vi "Begin.vi"() -> (0 "error out":errorcluster)   [LabVIEW 2013]
doc: "Called before other user functions, this VI is expected to open initial I/O refnums, load in file data, and do all program initialization. Notice that the <B>error out</B> terminal is simply used for data flow. Wiring it to other structures or subVIs ensures that this VI runs first."
uses:
  <vilib>/Rock Robotics/WPI/DriverStation/WPI_DriverStationRobotMode2.ctl
  <vilib>/Rock Robotics/WPI/Joystick/WPI_JoystickDeviceEnum.ctl
  <vilib>/Rock Robotics/WPI/SafetyOutput/WPI_SafetyOutputConfigMenu.ctl
  <vilib>/Rock Robotics/SystemInterfaces/DIO/FPGA_DIOPWMChannel.ctl
  Robot Global Data.vi
  <vilib>/Utility/config.llb/Read Key (Double).vi
  <vilib>/Utility/config.llb/Read Key (String).vi
  <vilib>/Rock Robotics/WPI/RobotDrive/WPI_RobotDriveOpen2MotorWithJaguar.vi
  <vilib>/Rock Robotics/WPI/MotorControl/WPI_MotorControlOpen Jaguar.vi
  <vilib>/Rock Robotics/SystemInterfaces/Typedef/FPGA_TypedefDigitalModule.ctl
  <vilib>/Rock Robotics/WPI/CAN/Jaguar/SubVIs/WPI_CANJaguar_ControlMode.ctl
  <vilib>/Rock Robotics/WPI/MotorControl/WPI_MotorControlOpenCANJaguar.vi
  <vilib>/Utility/config.llb/NI_LVConfig.lvlib
  <vilib>/Rock Robotics/WPI/Solenoid/WPI_SolenoidChannel.ctl
  <vilib>/Rock Robotics/SystemInterfaces/DIO/FPGA_DIOChannel.ctl
  <vilib>/Rock Robotics/SystemInterfaces/DIO/FPGA_DIORelayChannel.ctl
  <vilib>/Rock Robotics/WPI/Solenoid/WPI_SolenoidOpenSingle.vi
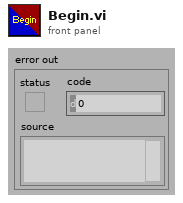
[diagram p1: front panel]
types:
  T1 = typedef "FPGA_DIOPWMChannel.ctl" = enum8{"PWM 1", "PWM 2", "PWM 3", "PWM 4", "PWM 5", "PWM 6", "PWM 7", "PWM 8", "PWM 9", "PWM 10", "Invalid"}
  T2 = typedef "WPI_SafetyOutputConfigMenu.ctl" = enum16{"Enable", "Disable"}
  T3 = typedef "WPI_JoystickDeviceEnum.ctl" = enum16{"USB 1", "USB 2", "USB 3", "USB 4", "Kinect 1", "Kinect 2"}
  T4 = cluster{"Left Motor Positions":cluster{"Low Extreme - 0 Degrees":dbl, "High Extreme - 180 Degrees":dbl}, "Right Motor Positions":cluster{"Low Extreme - 0 Degrees":dbl, "High Extreme - 180 Degrees":dbl}}
  T5 = cluster{"Low Extreme - 0 Degrees":dbl, "High Extreme - 180 Degrees":dbl}
  T6 = typedef "WPI_DriverStationRobotMode2.ctl" = enum16{"Autonomous Disabled", "Autonomous Enabled", "Teleop Disabled", "Teleop Enabled", "Timeout", "Finish", "Test Disabled", "Test Enabled"}
  T7 = typedef "NI_LVConfig.lvlib/Config Data RefNum.ctl" = refnum<k1>
  T8 = typedef "WPI_RobotDriveDevRef.ctl" = cluster{"DevStatus":errorcluster, "Motors[]":T9[], "Square Inputs":bool, "Max Output":dbl, "Isochronous":bool}
  T9 = typedef "WPI_MotorControlDeviceRef.ctl" = cluster{"DeviceStatus":errorcluster, "Type":enum16{"PWM", "CAN"}, "PWM":cluster{"Digital Module":T10, "PWM Channel":T1, "DeadBand":T11}, "CAN":cluster{"Device Number":u8, "Control Mode":T12, "Semaphore":T13, "Max Vout":dbl}, "Invert":bool, "TransformRef":T14, "InvTransformRef":T14}
  T10 = typedef "FPGA_TypedefDigitalModule.ctl" = enum16{"Digital Module 1", "Digital Module 2"}
  T11 = typedef "WPI_PWMDeadband.ctl" = cluster{"Name":string, "maxPositivePwm":i32, "minPositivePwm":i32, "centerPwm":i32, "maxNegativePwm":i32, "minNegativePwm":i32, "angularRange":u16}
  T12 = typedef "WPI_CANJaguar_ControlMode.ctl" = enum8{"Percent VBus", "Current", "Speed", "Position", "Voltage"}
  T13 = typedef "Semaphore RefNum" = refnum<k1>
  T14 = typedef "WPI_PWMTransform_ConPane.ctl" = refnum<vi>
  T15 = typedef "FPGA_DIORelayChannel.ctl" = enum8{"Relay 1", "Relay 2", "Relay 3", "Relay 4", "Relay 5", "Relay 6", "Relay 7", "Relay 8", "Invalid"}
  T16 = typedef "FPGA_DIOChannel.ctl" = enum8{"DIO 1", "DIO 2", "DIO 3", "DIO 4", "DIO 5", "DIO 6", "DIO 7", "DIO 8", "DIO 9", "DIO 10", "DIO 11", "DIO 12", "DIO 13", "DIO 14", "Invalid"}
  T17 = typedef "WPI_SolenoidChannel.ctl" = enum8{"Solenoid 1", "Solenoid 2", "Solenoid 3", "Solenoid 4", "Solenoid 5", "Solenoid 6", "Solenoid 7", "Solenoid 8", "Invalid"}
  T18 = typedef "WPI_SolenoidDevRef.ctl" = cluster{"DevStatus":errorcluster, "Solenoid Module":T19, "Forward Solenoid Channel":T17, "Reverse Solenoid Channel":T17}
  T19 = typedef "FPGA_TypedefSolenoidModule.ctl" = enum16{"Solenoid Module 1", "Solenoid Module 2"}
  T20 = typedef "WPI_CompressorDevRef.ctl" = cluster{"DevStatus":errorcluster, "DigitalInputDevRef":T21, "RelayDevRef":T22}
  T21 = typedef "WPI_DigitalInputDevRef.ctl" = cluster{"DevStatus":errorcluster, "DIO Channel":T16, "Digital Module":T10}
  T22 = typedef "WPI_RelayDevRef.ctl" = cluster{"DevStatus":errorcluster, "Relay Channel":T15, "Digital Module":T10, "Relay Direction":T23}
  T23 = typedef "WPI_RelayDirection.ctl" = enum16{"Both directions", "Forward only", "Reverse only"}
  T24 = typedef "WPI_JoystickDevRef.ctl" = cluster{"Device":T3}
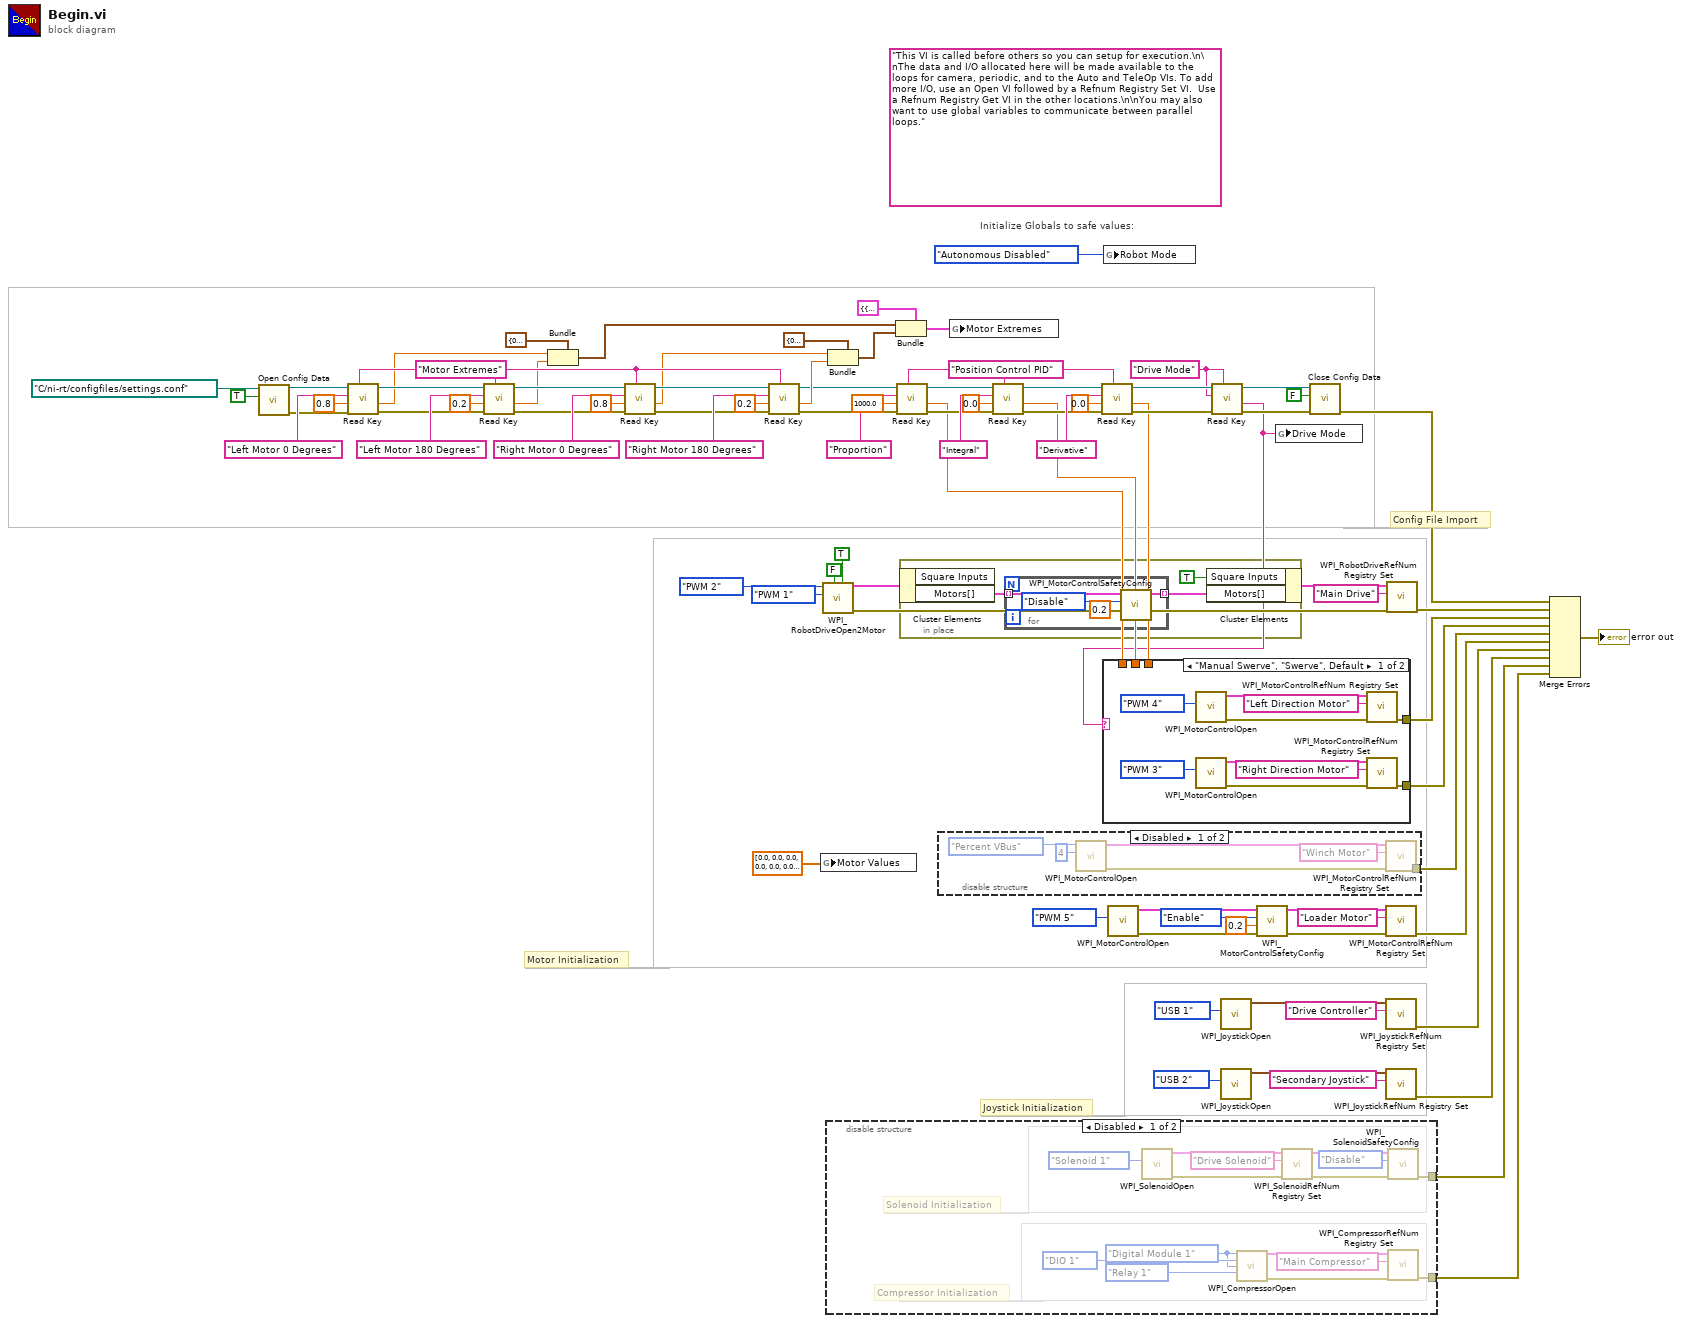
[diagram p0: block diagram]
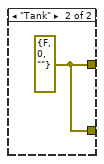
[diagram p4: hidden frame]
diagram:
  w25 = "Drive Mode" ("section")
  w54 = "Position Control PID" ("section")
  w68 = "Motor Extremes" ("section")
  (unwired) "This VI is called before others so you can setup for execution.\n\nThe data and I/O allocated here will be made available to the loops for camera, periodic, and to the Auto and TeleOp VIs. To add more I/O, use an Open VI followed by a Refnum Registry Set VI.  Use a Refnum Registry Get VI in the other locations.\n\nYou may also want to use global variables to communicate between parallel loops."
  # "Config File Import"
  # "Joystick Initialization"
  # "Motor Initialization"
  # "Initialize Globals to safe values:"
  n1 = call <vilib>:"Open Config Data.vi"("create file if necessary (T)"=TRUE, "configuration file path"=path "C:/ni-rt/configfiles/settings.conf") -> ("error out"=w32:errorcluster, "refnum"=w81:T7)  [unwired: 7 in, 1 out]
  n2 = call-poly <vilib>:"Read Key.vi"("section"=w68, "error in (no error)"=w32, "default value"=0.8, "key"="Left Motor 0 Degrees", "refnum"=w81) -> ("error out"=w33:errorcluster, "value"=w53:dbl, "refnum out"=w76:T7)  [unwired: 3 in, 1 out]
  n3 = call-poly <vilib>:"Read Key.vi"("section"=w68, "error in (no error)"=w33, "default value"=0.2, "key"="Left Motor 180 Degrees", "refnum"=w76) -> ("error out"=w34:errorcluster, "value"=w52:dbl, "refnum out"=w70:T7)  [unwired: 3 in, 1 out]
  n4 = Bundle(cluster=T5 {"Low Extreme - 0 Degrees"=0.0, "High Extreme - 180 Degrees"=0.0} ("Left Motor Positions"), "Low Extreme - 0 Degrees"=w53, "High Extreme - 180 Degrees"=w52) -> (w63:T5)
  n5 = call-poly <vilib>:"Read Key.vi"("section"=w68, "error in (no error)"=w34, "default value"=0.8, "key"="Right Motor 0 Degrees", "refnum"=w70) -> ("error out"=w35:errorcluster, "value"=w51:dbl, "refnum out"=w71:T7)  [unwired: 3 in, 1 out]
  n6 = call-poly <vilib>:"Read Key.vi"("section"=w68, "error in (no error)"=w35, "default value"=0.2, "key"="Right Motor 180 Degrees", "refnum"=w71) -> ("error out"=w36:errorcluster, "value"=w50:dbl, "refnum out"=w49:T7)  [unwired: 3 in, 1 out]
  n7 = global write "Robot Global Data.vi" "Motor Values"(dbl[] [0.0, 0.0, 0.0, 0.0, 0.0, 0.0, 0.0, 0.0]) -> ()
  n8 = call-poly <vilib>:"WPI_RobotDriveOpen2Motor.vi"("Right Motor Inverted"=TRUE, "Left Motor Inverted"=FALSE, "Right Motor"=FPGA_DIOPWMChannel."PWM 1", "Left Motor"=FPGA_DIOPWMChannel."PWM 2") -> ("error out"=w39:errorcluster, "RobotDriveDevRef"=w47:T8)  [unwired: 6 in]
  n9 = disable-structure shown="Disabled" {
    disable-tunnel: [w95 _] -> w23
    disable-tunnel: [w94 _] -> w19
    frame Disabled {
      w89 = FPGA_TypedefDigitalModule."Digital Module 1" ("Pressure Switch Digital Module (Module 1)")
      # "Compressor Initialization"
      # "Solenoid Initialization"
      n10 = call-poly <vilib>:"WPI_SolenoidOpen.vi"("Solenoid Channel"=WPI_SolenoidChannel."Solenoid 1") -> ("error out"=w101:errorcluster, "SolenoidDevRef"=w102:T18)  [unwired: 9 in]
      n11 = call <vilib>:"WPI_CompressorOpen.vi"("Pressure Switch Digital Module (Module 1)"=w89, "Pressure Switch DIO Channel"=FPGA_DIOChannel."DIO 1", "Relay Digital Module (Module 1)"=w89, "Relay Channel"=FPGA_DIORelayChannel."Relay 1") -> ("CompressorDevRef"=w93:T20, "error out"=w88:errorcluster)  [unwired: 10 in]
      n12 = call <vilib>:"WPI_SolenoidRefNum Registry Set.vi"("error in (no error)"=w101, "refnum name"="Drive Solenoid", "SolenoidDevRef"=w102) -> ("error out"=w99:errorcluster, "SolenoidDevRef"=w100:T18)  [unwired: 7 in]
      n13 = call <vilib>:"WPI_SolenoidSafetyConfig.vi"("error in (no error)"=w99, "mode"=WPI_SafetyOutputConfigMenu."Disable", "SolenoidDevRef"=w100) -> ("error out"=w95:errorcluster)  [unwired: 7 in, 1 out]
      n14 = call <vilib>:"WPI_CompressorRefNum Registry Set.vi"("error in (no error)"=w88, "refnum name"="Main Compressor", "CompressorDevRef"=w93) -> ("error out"=w94:errorcluster)  [unwired: 7 in, 1 out]
    }
    frame Enabled {
    }
  }
  n15 = Bundle(cluster=T5 {"Low Extreme - 0 Degrees"=0.0, "High Extreme - 180 Degrees"=0.0} ("Right Motor Positions"), "Low Extreme - 0 Degrees"=w51, "High Extreme - 180 Degrees"=w50) -> (w64:T5)
  n16 = Bundle(cluster=T4 {"Left Motor Positions"={"Low Extreme - 0 Degrees"=0.0, "High Extreme - 180 Degrees"=0.0}, "Right Motor Positions"={"Low Extreme - 0 Degrees"=0.0, "High Extreme - 180 Degrees"=0.0}} ("Motor Extremes"), "Left Motor Positions"=w63, "Right Motor Positions"=w64) -> (w48:T4)
  n17 = call-poly <vilib>:"Read Key.vi"("section"=w54, "error in (no error)"=w36, "default value"=1000.0, "key"="Proportion", "refnum"=w49) -> ("error out"=w37:errorcluster, "value"=w16:dbl, "refnum out"=w58:T7)  [unwired: 3 in, 1 out]
  n18 = in-place {
    n19 = in-place-cluster #1(w47) -> ("Motors[]"=w104:T9[])  [unwired: 1 out]
    n20 = for {
      tunnel: w104 -> [w109] mode=indexing
      tunnel: [w108] -> w103 mode=indexing
      n21 = call <vilib>:"WPI_MotorControlSafetyConfig.vi"("timeout (s)"=0.2, "mode"=WPI_SafetyOutputConfigMenu."Disable", "MotorControlDevRef"=w109) -> ("MotorControlDevRef"=w108:T9)  [unwired: 7 in, 1 out]
    }
    n22 = in-place-cluster #1("Square Inputs"=TRUE, "Motors[]"=w103) -> (w46:T8)
  }
  n23 = disable-structure shown="Disabled" {
    disable-tunnel: [w110 _] -> w30
    frame Disabled {
      n24 = call-poly <vilib>:"WPI_MotorControlOpen.vi"("Device Number"=u8 4, "Control Mode"=WPI_CANJaguar_ControlMode."Percent VBus") -> ("error out"=w111:errorcluster, "MotorControlDeviceRef"=w112:T9)  [unwired: 8 in]
      n25 = call <vilib>:"WPI_MotorControlRefNum Registry Set.vi"("error in (no error)"=w111, "refnum name"="Winch Motor", "MotorControlDevRef"=w112) -> ("error out"=w110:errorcluster)  [unwired: 7 in, 1 out]
    }
    frame Enabled {
    }
  }
  n26 = global write "Robot Global Data.vi" "Motor Extremes"(w48) -> ()
  n27 = call-poly <vilib>:"Read Key.vi"("section"=w54, "error in (no error)"=w37, "default value"=0.0, "key"="Integral", "refnum"=w58) -> ("error out"=w38:errorcluster, "value"=w17:dbl, "refnum out"=w55:T7)  [unwired: 3 in, 1 out]
  n28 = call-poly <vilib>:"Read Key.vi"("section"=w54, "error in (no error)"=w38, "default value"=0.0, "key"="Derivative", "refnum"=w55) -> ("error out"=w28:errorcluster, "value"=w18:dbl, "refnum out"=w29:T7)  [unwired: 3 in, 1 out]
  n29 = global write "Robot Global Data.vi" "Robot Mode"(WPI_DriverStationRobotMode2."Autonomous Disabled" ("Robot Mode")) -> ()
  n30 = call-poly <vilib>:"WPI_MotorControlOpen.vi"("PWM Channel"=FPGA_DIOPWMChannel."PWM 5") -> ("error out"=w6:errorcluster, "MotorControlDeviceRef"=w9:T9)  [unwired: 9 in]
  n31 = call-poly <vilib>:"Read Key.vi"("section"=w25, "error in (no error)"=w28, "key"=w25, "refnum"=w29) -> ("error out"=w27:errorcluster, "value"=w13:string, "refnum out"=w26:T7)  [unwired: 4 in, 1 out]
  n32 = case shown="\"Manual Swerve\", \"Swerve\", Default" w13 {
    tunnel: [w120 w126] -> w15
    tunnel: [w121 w126] -> w14
    tunnel: w18 -> [_ _]
    tunnel: w17 -> [_ _]
    tunnel: w16 -> [_ _]
    frame "Manual Swerve", "Swerve", Default {
      n33 = call-poly <vilib>:"WPI_MotorControlOpen.vi"("PWM Channel"=FPGA_DIOPWMChannel."PWM 4") -> ("error out"=w119:errorcluster, "MotorControlDeviceRef"=w124:T9)  [unwired: 9 in]
      n34 = call-poly <vilib>:"WPI_MotorControlOpen.vi"("PWM Channel"=FPGA_DIOPWMChannel."PWM 3") -> ("error out"=w118:errorcluster, "MotorControlDeviceRef"=w123:T9)  [unwired: 9 in]
      n35 = call <vilib>:"WPI_MotorControlRefNum Registry Set.vi"("error in (no error)"=w119, "refnum name"="Left Direction Motor", "MotorControlDevRef"=w124) -> ("error out"=w120:errorcluster)  [unwired: 7 in, 1 out]
      n36 = call <vilib>:"WPI_MotorControlRefNum Registry Set.vi"("error in (no error)"=w118, "refnum name"="Right Direction Motor", "MotorControlDevRef"=w123) -> ("error out"=w121:errorcluster)  [unwired: 7 in, 1 out]
    }
    frame "Tank" {
      w126 = errorcluster {"status"=FALSE, "code"=0, "source"=""} ("error out")
    }
  }
  n37 = call <vilib>:"WPI_JoystickOpen.vi"("JoystickDevice"=WPI_JoystickDeviceEnum."USB 1") -> ("JoystickDevRef"=w42:T24)  [unwired: 10 in]
  n38 = call <vilib>:"WPI_JoystickOpen.vi"("JoystickDevice"=WPI_JoystickDeviceEnum."USB 2") -> ("JoystickDevRef"=w45:T24)  [unwired: 10 in]
  n39 = call <vilib>:"WPI_MotorControlSafetyConfig.vi"("error in (no error)"=w6, "timeout (s)"=0.2, "mode"=WPI_SafetyOutputConfigMenu."Enable", "MotorControlDevRef"=w9) -> ("error out"=w7:errorcluster, "MotorControlDevRef"=w8:T9)  [unwired: 6 in]
  n40 = global write "Robot Global Data.vi" "Drive Mode"(w13) -> ()
  n41 = call <vilib>:"Close Config Data.vi"("error in (no error)"=w27, "write file if changed (T)"=FALSE, "refnum"=w26) -> ("error out"=w31:errorcluster)  [unwired: 7 in, 1 out]
  n42 = call <vilib>:"WPI_MotorControlRefNum Registry Set.vi"("error in (no error)"=w7, "refnum name"="Loader Motor", "MotorControlDevRef"=w8) -> ("error out"=w20:errorcluster)  [unwired: 7 in, 1 out]
  n43 = call <vilib>:"WPI_JoystickRefNum Registry Set.vi"("refnum name"="Drive Controller", "JoystickDevRef"=w42) -> ("error out"=w21:errorcluster)  [unwired: 8 in, 1 out]
  n44 = call <vilib>:"WPI_JoystickRefNum Registry Set.vi"("refnum name"="Secondary Joystick", "JoystickDevRef"=w45) -> ("error out"=w22:errorcluster)  [unwired: 8 in, 1 out]
  n45 = call <vilib>:"WPI_RobotDriveRefNum Registry Set.vi"("error in (no error)"=w39, "refnum name"="Main Drive", "RobotDriveDevRef"=w46) -> ("error out"=w85:errorcluster)  [unwired: 7 in, 1 out]
  n46 = Merge Errors(w31, w85, w15, w14, w30, w20, w21, w22, w23, w19) -> (→"error out":errorcluster)
